vi "Query Weather Data.vi"(8 "Error In":errorcluster, 10 "Coordenates":T4 {"Longitude" format="%#_13g"; "Latitude" format="%#_13g"}, 11 "Open Weather Session In":refnum<class "Open Weather Session.lvclass">) -> (0 "Error Out":errorcluster, 2 "Weather Data":T1, 3 "Open Weather Session Out":refnum<class "Open Weather Session.lvclass">)   [LabVIEW 2019, in "Open Weather Session.lvclass"]
uses:
  Open Weather Session.lvclass
  Controls/Coordenates.ctl
  Controls/Weather Data.ctl
  Controls/Weather Sample Data.ctl
  Controls/Weather Description Data.ctl
  Accessors/REST Client/Get REST Client.vi
  Accessors/REST Client/Set REST Client.vi
  <vilib>/addons/_JKI.lib/REST Client/classes/REST Client/REST Client.lvclass
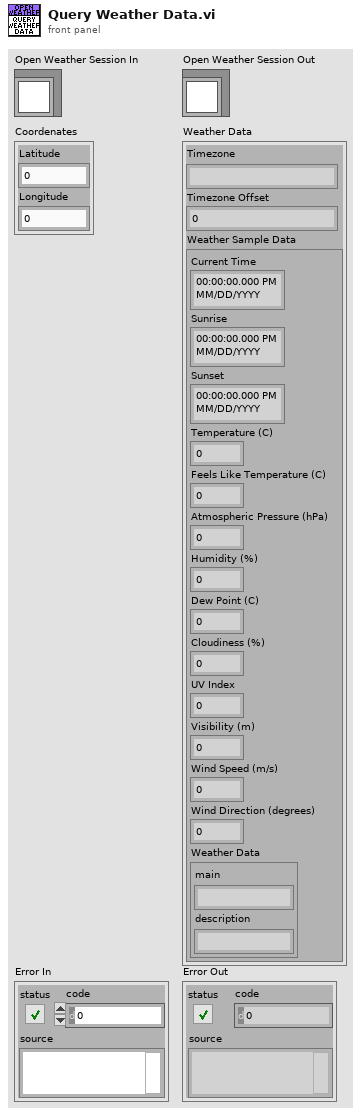
[diagram p1: front panel]
types:
  T1 = typedef "Open Weather Session.lvclass/Weather Data.ctl" = cluster{"Timezone":string, "Timezone Offset":dbl, "Weather Sample Data":T2}
  T2 = typedef "Open Weather Session.lvclass/Weather Sample Data.ctl" = cluster{"Current Time":timestamp, "Sunrise":timestamp, "Sunset":timestamp, "Temperature (C)":dbl, "Feels Like Temperature (C)":dbl, "Atmospheric Pressure (hPa)":dbl, "Humidity (%)":dbl, "Dew Point (C)":dbl, "Cloudiness (%)":dbl, "UV Index":dbl, "Visibility (m)":dbl, "Wind Speed (m/s)":dbl, "Wind Direction (degrees)":dbl, "Weather Data":T3}
  T3 = typedef "Open Weather Session.lvclass/Weather Description Data.ctl" = cluster{"main":string, "description":string}
  T4 = typedef "Open Weather Session.lvclass/Coordenates.ctl" = cluster{"Latitude":dbl, "Longitude":dbl}
  T5 = typedef "Open Weather Session.lvclass/Raw Weather Data.ctl" = cluster{"lat":dbl, "lon":dbl, "timezone":string, "timezone_offset":dbl, "current":T6}
  T6 = typedef "Open Weather Session.lvclass/Weather Sample Raw Data.ctl" = cluster{"dt":dbl, "sunrise":dbl, "sunset":dbl, "temp":dbl, "feels_like":dbl, "pressure":i32, "humidity":i32, "dew_point":dbl, "uvi":dbl, "clouds":i32, "visibility":i32, "wind_speed":dbl, "wind_deg":i32, "weather":T7[]}
  T7 = typedef "Open Weather Session.lvclass/Weather Description Raw Data.ctl" = cluster{"id":u32, "main":string, "description":string, "icon":string}
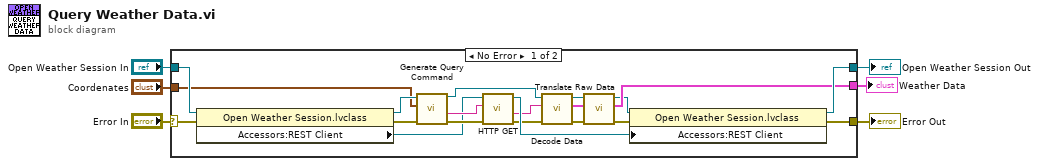
[diagram p0: block diagram]
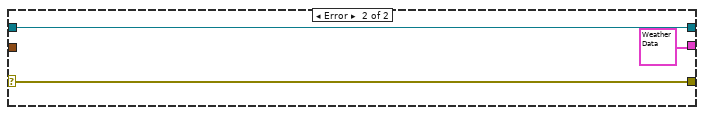
[diagram p2: hidden frame]
diagram:
  n1 = case shown="No Error" "Error In" {
    selector: "Error In" -> [w24 w28]
    tunnel: [w17 w28] -> w5
    tunnel: [w18 w29] -> w4
    tunnel: "Open Weather Session In" -> [w23 w29]
    tunnel: "Coordenates" -> [w16 _]
    tunnel: [w9 T1 {"Timezone"="", "Timezone Offset"=0.0, "Weather Sample Data"={"Current Time"=timestamp(0 s since 1904-01-01), "Sunrise"=timestamp(0 s since 1904-01-01), "Sunset"=timestamp(0 s since 1904-01-01), "Temperature (C)"=0.0, "Feels Like Temperature (C)"=0.0, "Atmospheric Pressure (hPa)"=0.0, "Humidity (%)"=0.0, "Dew Point (C)"=0.0, "Cloudiness (%)"=0.0, "UV Index"=0.0, "Visibility (m)"=0.0, "Wind Speed (m/s)"=0.0, "Wind Direction (degrees)"=0.0, "Weather Data"={"main"="", "description"=""}}} ("Weather Data")] -> w1
    frame No Error {
      n2 = property class="Open Weather Session.lvclass"(reference=w23, error in=w24) -> (reference out=w22:refnum<class "Open Weather Session.lvclass">, error out=w21:errorcluster, "Accessors:REST Client"=w20:refnum<class "REST Client.lvclass">)
      n3 = call "Generate Query Command.vi"("Error In"=w21, "Coordenates"=w16, "Open Weather Session In"=w22) -> ("Error Out"=w25:errorcluster, "Query Command"=w26:string, "Open Weather Session Out"=w14:refnum<class "Open Weather Session.lvclass">)  [unwired: 6 in]
      n4 = call-dynamic "HTTP GET.vi"("error in (no error)"=w25, "Path"=w26, "REST Client in"=w20) -> ("error out"=w13:errorcluster, "Response body"=w15:string, "REST Client out"=w19:refnum<class "REST Client.lvclass">)  [unwired: 3 in, 3 out]
      n5 = call "Decode Data.vi"("Error In"=w13, "Response String"=w15, "Open Weather Session In"=w14) -> ("Error Out"=w10:errorcluster, "Raw Weather Data"=w11:T5, "Open Weather Session Out"=w12:refnum<class "Open Weather Session.lvclass">)  [unwired: 6 in]
      n6 = call "Translate Raw Data.vi"("Error In"=w10, "Raw Weather Data"=w11, "Open Weather Session In"=w12) -> ("Error Out"=w7:errorcluster, "Weather Data"=w9:T1, "Open Weather Session Out"=w8:refnum<class "Open Weather Session.lvclass">)  [unwired: 6 in]
      n7 = property class="Open Weather Session.lvclass"(reference=w8, error in=w7, "Accessors:REST Client"=w19) -> (reference out=w18:refnum<class "Open Weather Session.lvclass">, error out=w17:errorcluster)
    }
    frame Error {
    }
  }
  "Error Out" <- w5
  "Open Weather Session Out" <- w4
  "Weather Data" <- w1
